vi "Get Value Between.vi"(9 "Y":dbl[](array[numeric]), 10 "X":dbl[](array[numeric]), 11 "input":dbl) -> (3 "output":dbl)   [LabVIEW 2016]
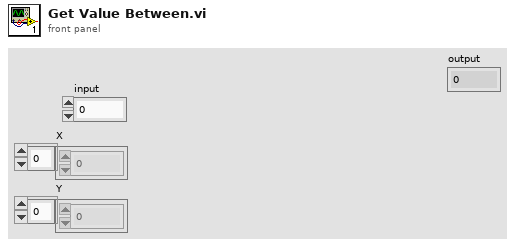
[diagram p1: front panel]
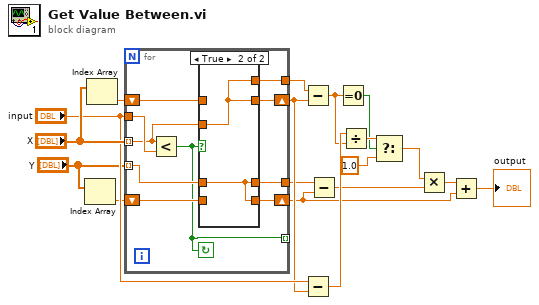
[diagram p0: block diagram]
diagram:
  n1 = Index Array(array="Y") -> (element=w12:dbl)  [unwired: 1 in]
  n2 = Index Array(array="X") -> (element=w17:dbl)  [unwired: 1 in]
  n3 = for {
    tunnel: "X" -> [w27] mode=indexing
    tunnel: "input" -> [w28]
    shift-right: [w26] -> w13
    shift-left: w17 -> [w25]
    tunnel: [w24] -> w16
    tunnel: "Y" -> [w20] mode=indexing
    shift-right: [w22] -> w7
    shift-left: w12 -> [w23]
    tunnel: [w21] -> w10
    tunnel: [w19] -> _ mode=indexing
    stop <- w19 continue-if-true
    n4 = Less?(x=w27, y=w28) -> (x < y?=w19:bool)
    n5 = case shown="True" w19 {
      tunnel: w27 -> [w31 w34]
      tunnel: [w32 w34] -> w26
      tunnel: w25 -> [w32 _]
      tunnel: [w31 w34] -> w24
      tunnel: [w30 w33] -> w22
      tunnel: w23 -> [w30 _]
      tunnel: [w29 w33] -> w21
      tunnel: w20 -> [w29 w33]
      frame False {
      }
      frame True {
      }
    }
  }
  n6 = Subtract(x=w16, y=w13) -> (x-y=w5:dbl)
  n7 = Subtract(x="input", y=w13) -> (x-y=w14:dbl)
  n8 = Subtract(x=w10, y=w7) -> (x-y=w9:dbl)
  n9 = Equal To 0?(x=w5) -> (x = 0?=w3:bool)
  n10 = Divide(x=w14, y=w5) -> (x/y=w4:dbl)
  n11 = Select(t=w4, s=w3, f=1.0) -> (s? t:f=w1:dbl)
  n12 = Multiply(x=w1, y=w9) -> (x*y=w8:dbl)
  n13 = Add(x=w8, y=w7) -> (x+y=→"output":dbl)
